vi "Helper SubVI - Compute Padding Zeroes.vi"(9 "config":T1={"new sample period"=0.0, "Timing Jitter"=enum."Interpolation", "first point location"=0.0, "prototype filter"={"h"=[], "Max Decimation"=1000}} {"prototype filter"."h" format="%#.6g"; "first point location" format="%#.6g"; "new sample period" format="%#.6g"}, 10 "anti-aliasing?":bool=TRUE, 11 "length of X":i32) -> (1 "length of Y (after padding zeroes)":i32, 2 "length of Y":i32, 3 "length of padding zeroes":i32)   [LabVIEW 2020]
doc: "Compute padding zeroes based on the formula defined on the block diagram of this VI."
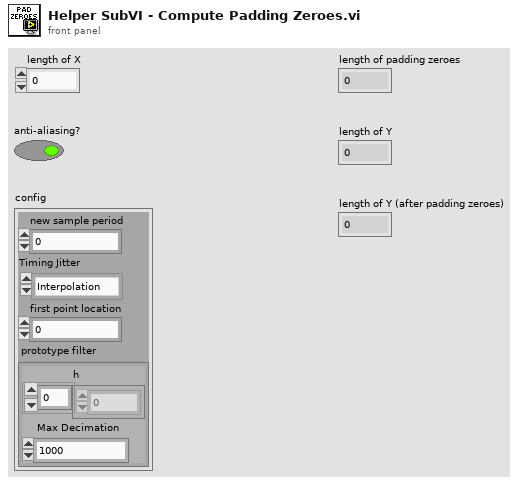
[diagram p1: front panel]
types:
  T1 = cluster{"new sample period":dbl, "Timing Jitter":enum32{"Interpolation", "Rounding"}, "first point location":dbl, "prototype filter":cluster{"h":dbl[], "Max Decimation":i32}}
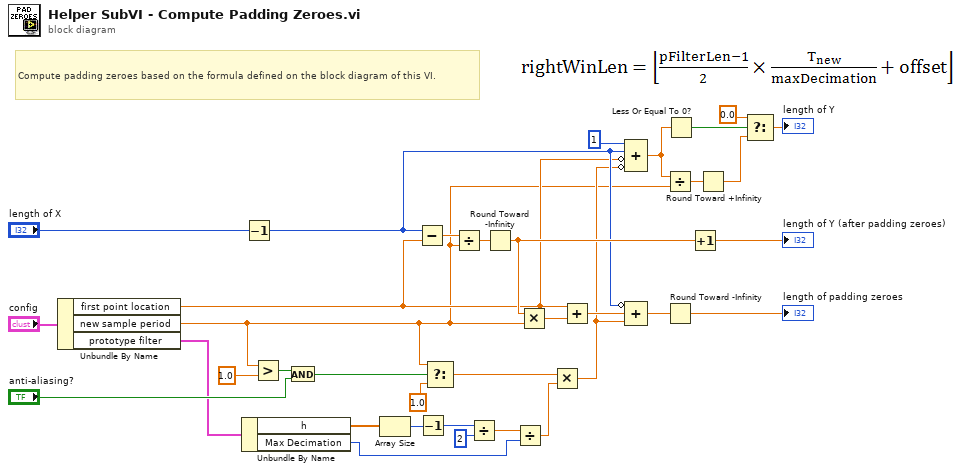
[diagram p0: block diagram]
diagram:
  # "Compute padding zeroes based on the formula defined on the block diagram of this VI."
  n1 = Unbundle By Name("config") -> ("first point location"=w9:dbl, "new sample period"=w7:dbl, "prototype filter"=w26:cluster{"h":dbl[], "Max Decimation":i32})
  n2 = Unbundle By Name(w26) -> ("h"=w25:dbl[], "Max Decimation"=w20:i32)
  n3 = Decrement(x="length of X") -> (x-1=w10:i32)
  n4 = Greater?(x=w7, y=1.0) -> (0:w13:bool)
  n5 = And(x=w13, y="anti-aliasing?") -> (x .and. y?=w16:bool)
  n6 = Array Size(array=w25) -> (size(s)=w24:i32)
  n7 = Subtract(x=w10, y=w9) -> (x-y=w29:dbl)
  n8 = Decrement(x=w24) -> (x-1=w23:i32)
  n9 = Select(t=w7, s=w16, f=1.0) -> (s? t:f=w14:dbl)
  n10 = Divide(x=w29, y=w7) -> (x/y=w28:dbl)
  n11 = Divide(x=w23, y=2) -> (x/y=w21:dbl)
  n12 = Round Toward -Infinity(1:w28) -> (0:w11:dbl)
  n13 = Divide(x=w21, y=w20) -> (x/y=w19:dbl)
  n14 = Multiply(x=w11, y=w7) -> (x*y=w27:dbl)
  n15 = Multiply(x=w14, y=w19) -> (x*y=w8:dbl)
  n16 = Add(x=w9, y=w27) -> (x+y=w12:dbl)
  n17 = Compound Arithmetic op=ADD(1 ("value"), w10, invert w9, invert w8) -> (w4:dbl)
  n18 = Compound Arithmetic op=ADD(invert w10, w12, w8) -> (w18:dbl)
  n19 = Divide(x=w4, y=w7) -> (x/y=w3:dbl)
  n20 = Round Toward -Infinity(1:w18) -> (0:→"length of padding zeroes":dbl)
  n21 = Less Or Equal To 0?(x=w4) -> (x <= 0?=w6:bool)
  n22 = Increment(x=w11) -> (x+1=→"length of Y (after padding zeroes)":dbl)
  n23 = Round Toward +Infinity(x=w3) -> (ceil(x): smallest int >= x=w2:dbl)
  n24 = Select(t=0.0, s=w6, f=w2) -> (s? t:f=→"length of Y":dbl)
